vi "util.procs.find-by-name.vi"(6 "isRequired(T)":bool=TRUE, 8 "error in":errorcluster, 10 "ProcName in":string, 11 "Procs in":cluster{"Procedure":variant[]}[](array[cluster])) -> (0 "error out":errorcluster, 1 "ProcHead":variant, 2 "Found?":bool, 3 "procIndex":i32, 4 "Proc Path":string, 5 "Found Proc":cluster{"Procedure":variant[]})   [LabVIEW 2024]
uses:
  controls/typeProcVarientName.ctl
  controls/typeEngErrorCodes.ctl
  Polymorphics/variantCtrlString.vi
  <vilib>/Utility/error.llb/Clear Errors.vi
panel:
  out "Array":string[](array[string])
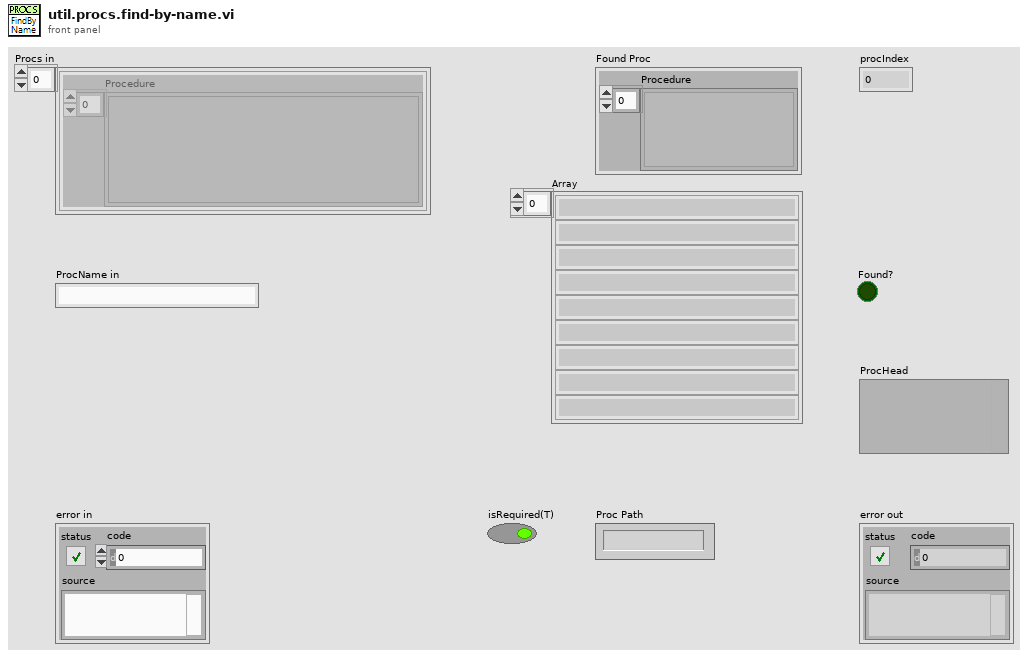
[diagram p1: front panel]
types:
  T1 = typedef "typeProcVarientName.ctl" = enum16{"procNameID", "procModuleID", "procPath", "procIsRunning", "procIndex", "procModule", "procRegisterNumeric", "procRegisterString", "procReport", "procReportPrev", "procCLK", "procStepPointer", "procType"}
  T2 = typedef "typeEngErrorCodes.ctl" = u16
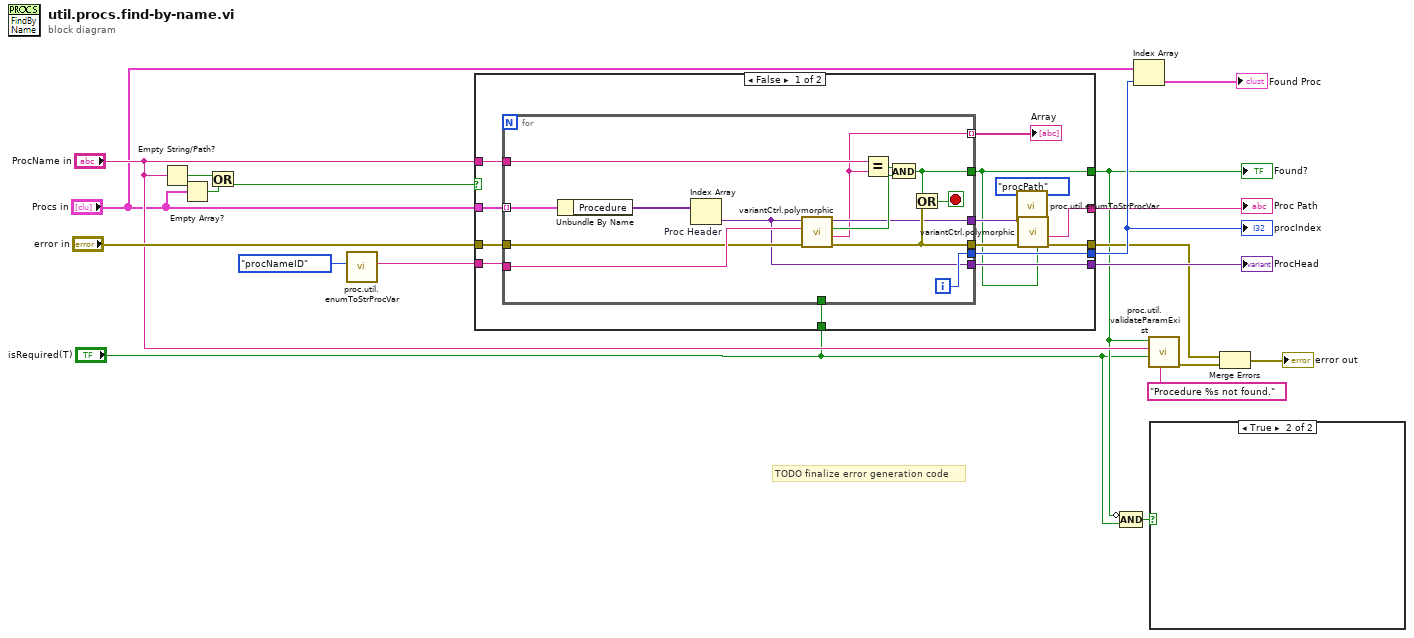
[diagram p0: block diagram]
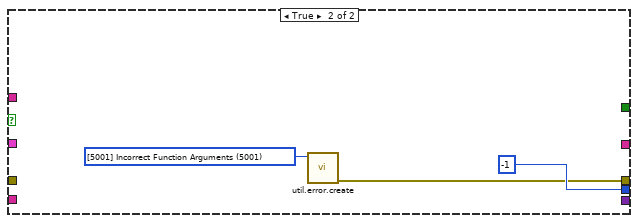
[diagram p3: hidden frame]
diagram:
  # "TODO finalize error generation code"
  n1 = Empty String/Path?(string/path="ProcName in") -> (empty?=w16:bool)
  n2 = Empty Array?(array="Procs in") -> (empty?=w15:bool)
  n3 = Or(x=w16, y=w15) -> (x .or. y?=w14:bool)
  n4 = call "proc.util.enumToStrProcVar.vi"("Proc var"=typeProcVarientName."procNameID" ("name")) -> ("String"=w18:string)  [unwired: 10 in]
  n5 = case shown="False" w14 {
    tunnel: [w34 -1] -> w9
    tunnel: "ProcName in" -> [w33 _]
    tunnel: w18 -> [w32 _]
    tunnel: [w20 _] -> w3
    tunnel: "error in" -> [w31 _]
    tunnel: [w23 w49] -> w4
    tunnel: "Procs in" -> [w30 _]
    tunnel: [w29 _] -> w10
    tunnel: [w26 _] -> w6
    tunnel: "isRequired(T)" -> [w21 _]
    frame False {
      n6 = for {
        tunnel: w30 -> [w48] mode=indexing
        tunnel: w33 -> [w47]
        tunnel: [w42] -> w20
        tunnel: [w44] -> w34
        tunnel: w32 -> [w43]
        tunnel: [w41] -> w24
        tunnel: w31 -> [w38]
        tunnel: [w37] -> w29
        tunnel: [w36] -> w25
        tunnel: [w35] -> w22 mode=indexing
        tunnel: w21 -> [_]
        i -> [w44]
        stop <- w40 stop-if-true
        n7 = Unbundle By Name(w48) -> ("Procedure"=w39:variant[])
        n8 = Index Array "Proc Header"(array=w39) -> (element=w37:variant)  [unwired: 1 in]
        n9 = call-poly "variantCtrl.polymorphic.vi"("error in"=w38, "name in"=w43, "Step in"=w37) -> ("error out"=w41:errorcluster, "String Value"=w35:string, "isFound?"=w46:bool, "Step out"=w36:variant)  [unwired: 5 in]
        n10 = Equal?(x=w47, y=w35) -> (x = y?=w45:bool)
        n11 = And(x=w45, y=w46) -> (x .and. y?=w42:bool)
        n12 = Or(x=w42, y=w41) -> (x .or. y?=w40:bool)
      }
      "Array" <- w22
      n13 = call "proc.util.enumToStrProcVar.vi"("Proc var"=typeProcVarientName."procPath" ("name")) -> ("String"=w28:string)  [unwired: 10 in]
      n14 = call-poly "variantCtrl.polymorphic.vi"("isRequired (T)"=w20, "error in"=w24, "name in"=w28, "Step in"=w25) -> ("error out"=w23:errorcluster, "String Value"=w26:string)  [unwired: 4 in, 2 out]
    }
    frame True {
      w50 = T2 5001 items=["[5000] Missing Function Arguments"=5000, "[5001] Incorrect Function Arguments"=5001] ("Ring")
      n15 = call "util.error.create.vi"("Ring"=w50) -> ("error out"=w49:errorcluster)  [unwired: 9 in, 1 out]
    }
  }
  "Found?" <- w3
  "ProcHead" <- w10
  "Proc Path" <- w6
  "procIndex" <- w9
  n16 = Compound Arithmetic op=AND(invert w3, "isRequired(T)") -> (w2:bool)
  n17 = Index Array(array="Procs in", index=w9) -> (element=→"Found Proc":cluster{"Procedure":variant[]})
  n18 = call "proc.util.validateParamExist.vi"("format string"="Procedure %s not found.", "isRequired"="isRequired(T)", "Param Label"="ProcName in", "isFound"=w3) -> ("error out"=w12:errorcluster)  [unwired: 7 in]
  n19 = case shown="True" w2 {
    frame False {
    }
    frame True {
    }
  }
  n20 = Merge Errors(w4, w12) -> (→"error out":errorcluster)
